vi "Read Bool.vi"(8 "error in (no error)":errorcluster, 10 "Start address":string, 11 "MelsecTCP in":refnum<class "Abs Controler.lvclass">) -> (0 "error out":errorcluster, 2 "Data":bool, 3 "MelsecTCP out":refnum<class "Abs Controler.lvclass">)   [LabVIEW 2020, in "HslCommunication.lvlib" / "Abs Controler.lvclass"]
uses:
  Abs Controler.lvclass
  E:/Git/Libraries/develop/HslCommunication/_Dependenciecs/HslCommunication.dll
  _Dependenciecs/HslCommunication.dll
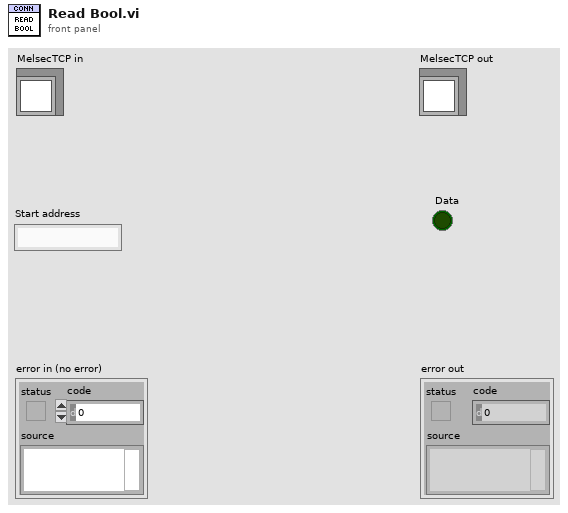
[diagram p1: front panel]
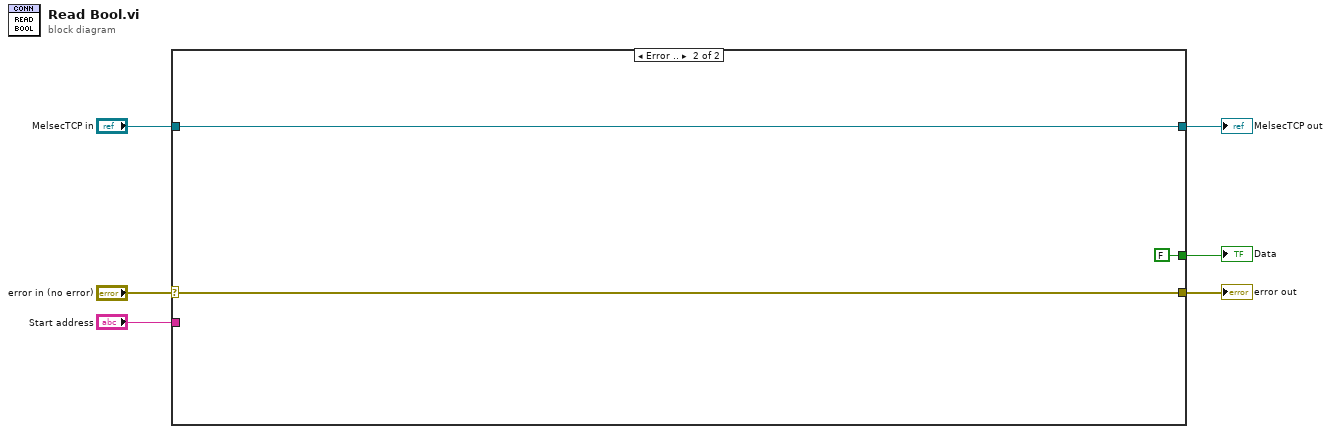
[diagram p0: block diagram]
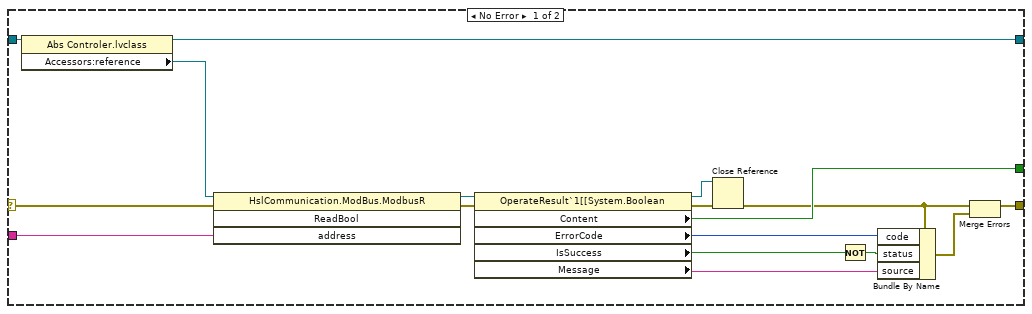
[diagram p2: hidden frame]
diagram:
  n1 = case shown="Error .." "error in (no error)" {
    selector: "error in (no error)" -> [w12 w26]
    tunnel: "MelsecTCP in" -> [w23 w25]
    tunnel: [w14 w25] -> w2
    tunnel: "Start address" -> [w13 _]
    tunnel: [w20 w26] -> w3
    tunnel: [w21 FALSE ("Content")] -> w1
    frame No Error {
      n2 = property class="Abs Controler.lvclass"(reference=w23) -> (reference out=w14:refnum<class "Abs Controler.lvclass">, "Accessors:reference"=w22:refnum<k24>)  [unwired: 1 in, 1 out]
      n3 = invoke class="HslCommunication.ModBus.ModbusR" method="ReadBool"(reference=w22, error in=w12, "address"=w13) -> (error out=w10:errorcluster, "ReadBool"=w8:refnum<k24>)  [unwired: 1 in, 2 out]
      n4 = property class="OperateResult`1[[System.Boolean"(reference=w8, error in=w10) -> (reference out=w7:refnum<k24>, error out=w9:errorcluster, "Content"=w21:bool, "ErrorCode"=w19:i32, "IsSuccess"=w18:bool, "Message"=w17:string)
      n5 = Close Reference(reference=w7, error in (no error)=w9) -> (error out=w16:errorcluster)
      n6 = Not(x=w18) -> (.not. x?=w11:bool)
      n7 = Bundle By Name(cluster=w16, "code"=w19, "status"=w11, "source"=w17) -> (w15:errorcluster)
      n8 = Merge Errors(w16, w15) -> (w20:errorcluster)
    }
    frame Error {
    }
  }
  "error out" <- w3
  "MelsecTCP out" <- w2
  "Data" <- w1
